vi "Multiprocessing_VI.vi"() -> ()   [LabVIEW 2022 SP3]
uses:
  <vilib>/Analysis/baseanly.llb/Mean (DBL).vi
  <vilib>/DAQmx/read.llb/DAQmx Read (Analog 1D Wfm NChan NSamp).vi
  STOP_GLOBAL.vi
  <vilib>/DAQmx/configure/timing.llb/DAQmx Timing (Sample Clock).vi
  <vilib>/addons/control/pid/pid.llb/PID Gain Schedule (DBL).vi
  <vilib>/DAQmx/miscellaneous.llb/DAQmx Fill In Error Info.vi
  <resource>/objmgr/daqmx.rc
  <vilib>/addons/control/pid/NI_PID_pid.lvlib
  <vilib>/Analysis/NI_AALBase.lvlib
panel:
  out "Angle Command":dynamicdata(graph)
  in  "Ignition":bool
  in  "Stepper Voltage":ext format="%_3g"
  out "Chamber Pressure LocalVar":dynamicdata(graph)
  out "PID gains out":T1={"proportional gain (Kc)"=1.0, "integral time (Ti, min)"=0.01, "derivative time (Td, min)"=0.0} {"derivative time (Td, min)" format="%.3f"; "integral time (Ti, min)" format="%.5f"; "proportional gain (Kc)" format="%.3f"}
  out "Process Variable vs Setpoint":dynamicdata(graph)
  out "Output":dbl(slide)=30.8641975308642 scale=0.0..5.067 scale format="%.1f"
  in  "Automatic":bool=TRUE
  out "Servo Voltage":dbl[](array[numeric])
  in  "SP":dbl
  in  "MV":dbl(slide)=30.8641975308642 scale=0.0..5.067 scale format="%.1f"
  in  "Stop All":bool
  out "x*y 2":dbl
  out "AI7":dynamicdata(graph)
  out "Time":dbl
  out "Inlet Thermocouple":cluster{dbl[], dbl[]}(graph)
  out "Inlet Thermocouple":dynamicdata(graph)
  out "Flow Meter Thermocouple":dynamicdata(graph)
  out "Supply P. Thermocouple":cluster{dbl[], dbl[]}(graph)
  out "Flow Meter Thermocouple":cluster{dbl[], dbl[]}(graph)
  out "Supply P. Thermocouple":dynamicdata(graph)
  out "Thrust 3":cluster{dbl[], dbl[]}(graph)
  out "Thrust 2":cluster{dbl[], dbl[]}(graph)
  out "Rocket Thrust":cluster{dbl[], dbl[]}(graph)
  out "LC3":dynamicdata(graph)
  out "LC2":dynamicdata(graph)
  out "Rocket Thrust LC1":dynamicdata(graph)
  out "Waiting \nfor Start":bool=TRUE
  in  "Start VI":bool
  out "SampClk.Rate":dbl
  in  "Sample Number":i32=100
  in  "Channel Control":bool[](array[boolean])
  in  "Rate":dbl=1000.0 format="%0.2f"
  out "AI7":cluster{dbl[], dbl[]}(graph)
  out "Vol Flow L/min":dynamicdata(graph)
  out "Process Variable vs Setpoint":cluster{dbl[], dbl[]}[](graph)
  in  "Filename":path=path "C:/1. Rocket Research Project/CollectedData/Plots/TestingData.lvm"
  in  "PID gain schedule":T2(array[cluster])=[{"PID gains"={"proportional gain (Kc)"=1.0, "integral time (Ti, min)"=0.01, "derivative time (Td, min)"=0.0}, "max value"=100.0}] {"max value" format="%.2f"; "PID gains"."derivative time (Td, min)" format="%.3f"; "PID gains"."integral time (Ti, min)" format="%.3f"; "PID gains"."proportional gain (Kc)" format="%.3f"}
  in  "Collect?":bool=TRUE caption="Enable"
  out "Vol Flow":cluster{dbl[], dbl[]}(graph)
  out "Chamber Pressure":cluster{dbl[], dbl[]}(graph)
  out "Inlet Pressure":cluster{dbl[], dbl[]}(graph)
  out "Line Pressure":cluster{dbl[], dbl[]}(graph)
  out "Supply Pressure":cluster{dbl[], dbl[]}(graph)
  out "Supply Pressure":dynamicdata(graph)
  out "Inlet Pressure":dynamicdata(graph)
  out "Line Pressure":dynamicdata(graph)
  out "Chamber Pressure PSI":dynamicdata(graph)
  out "Output Clock Rate":dbl
  out "x*y":i32
  out "error out":errorcluster
  out "Iterations":i32
  out "AI6":dynamicdata(graph)
  out "P.T. 5":dynamicdata(graph)
  # "Pressure Channels"
  # "Temperature Channels"
  # "Thrust Channels"
  # "DAQ Configuration"
  # "AI 0 - Supply Pressure"
  # "AI 1 - Flow Meter Pressure"
  # "AI 2 - Inlet Pressure"
  # "AI 3 - Chamber Pressure"
  # "AI 4 - Differential Pressure"
  # "AI 5 - Volumetric Flow"
  # "AI 6"
  # "AI 7"
  # "Load Cell 1 Right"
  # "Load Cell 2 Left"
  # "Thrust Channel 3"
  # "TC1 - Supply P. Thermocouple"
  # "TC2 - Flow Meter Thermocouple"
  # "TC3 - Inlet Thermocouple"
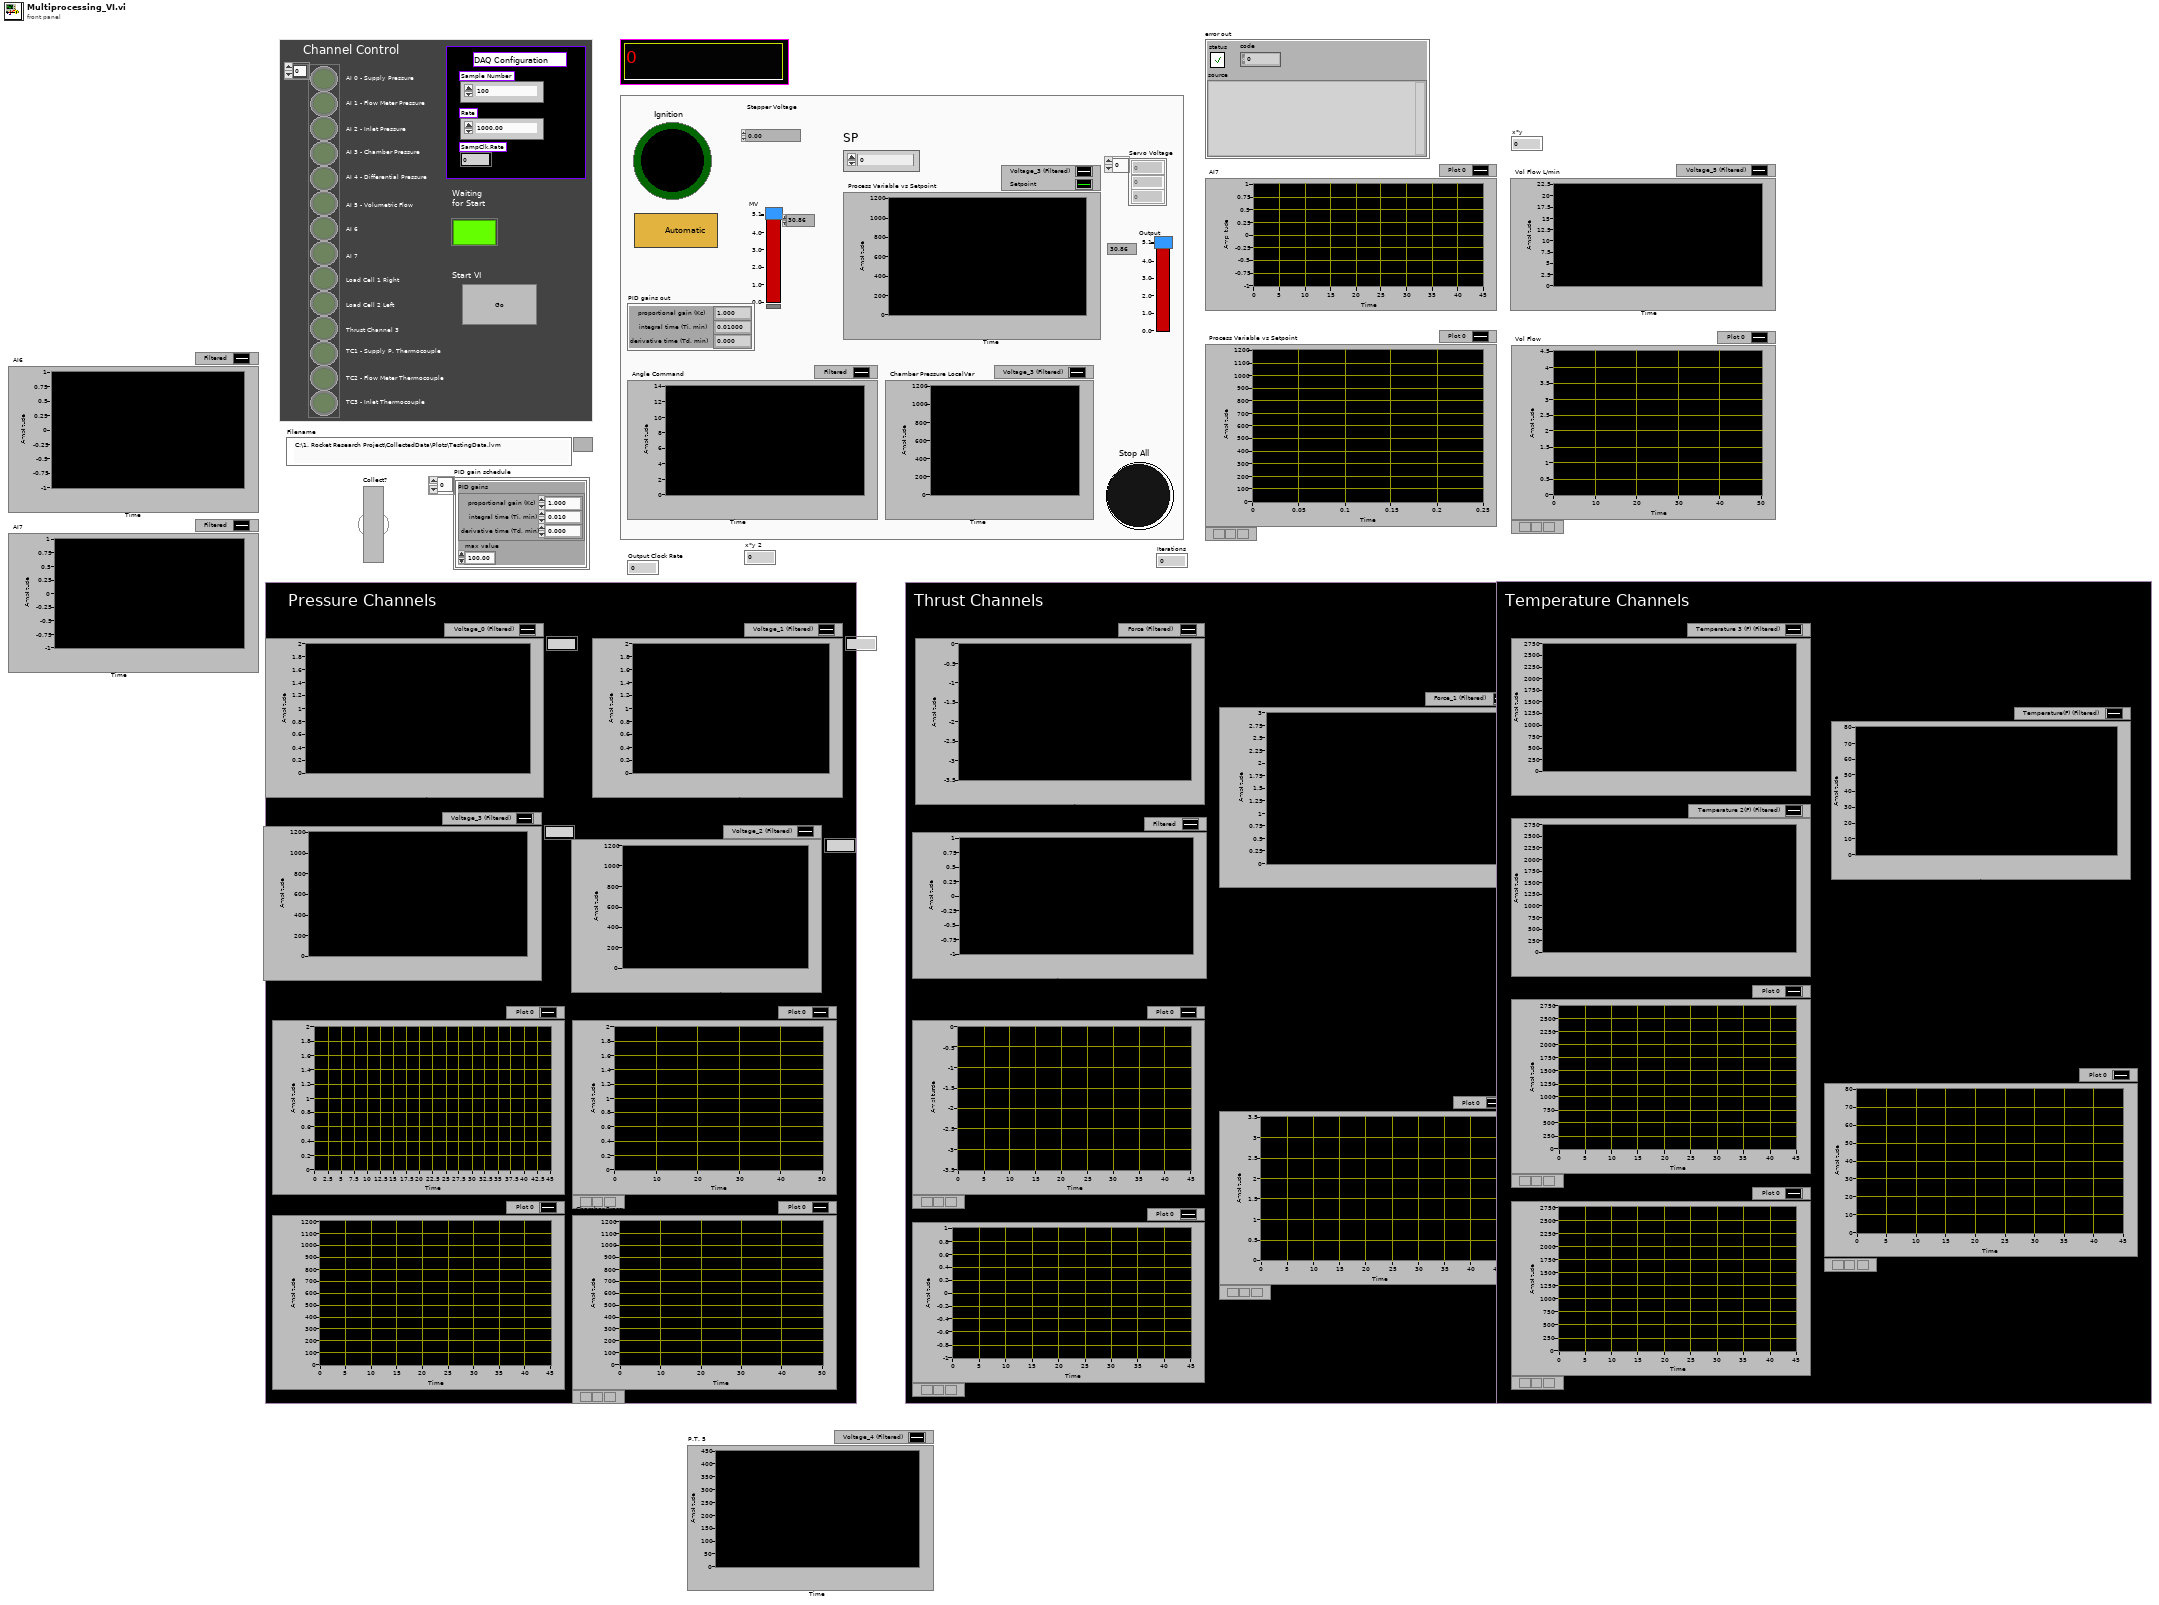
[diagram p1: front panel]
types:
  T1 = cluster{"proportional gain (Kc)":dbl, "integral time (Ti, min)":dbl, "derivative time (Td, min)":dbl}
  T2 = cluster{"PID gains":cluster{"proportional gain (Kc)":dbl, "integral time (Ti, min)":dbl, "derivative time (Td, min)":dbl}, "max value":dbl}[]
  T3 = cluster{"PID gains":cluster{"Kc":dbl, "Ti":dbl, "Td":dbl}, "max value":dbl}[]
  T4 = cluster{"Modulus":dbl, "Number of\nComplete Cycles":dbl}
  T5 = cluster{"Dynamic Data":dynamicdata, "Dynamic Data":dynamicdata, "Dynamic Data":dynamicdata, "Dynamic Data":dynamicdata, "Dynamic Data":dynamicdata, "Dynamic Data":dynamicdata, "Dynamic Data":dynamicdata, "Dynamic Data":dynamicdata, "Dynamic Data":dynamicdata, "Dynamic Data":dynamicdata, "Dynamic Data":dynamicdata, "Dynamic Data":dynamicdata, "Dynamic Data":dynamicdata, "Dynamic Data":dynamicdata}
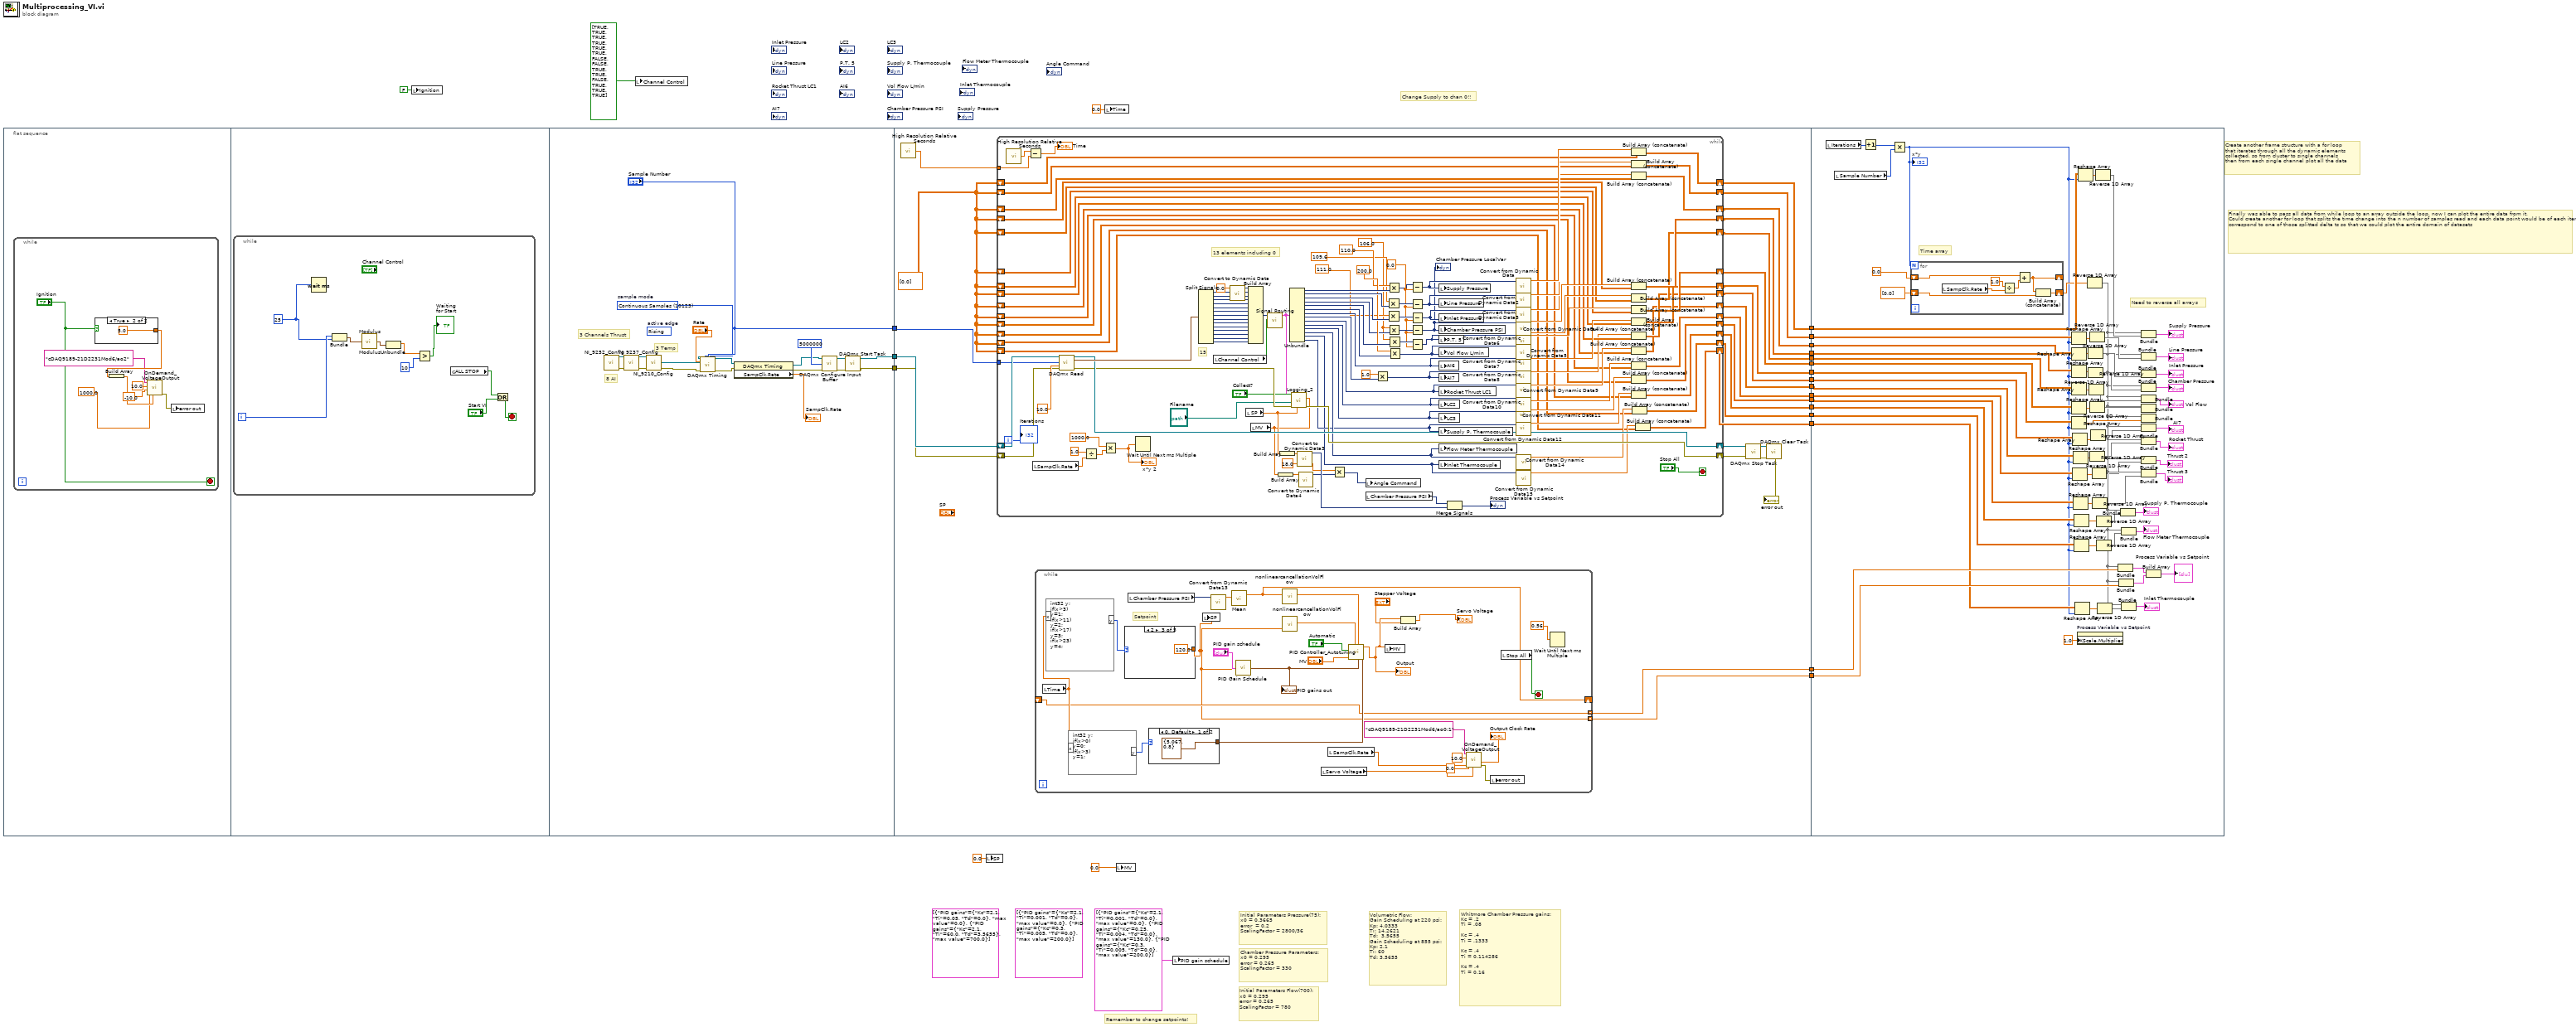
[diagram p0: block diagram]
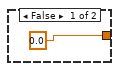
[diagram p2: hidden frame]
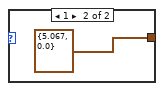
[diagram p3: hidden frame]
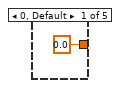
[diagram p4: hidden frame]
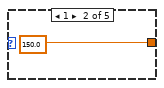
[diagram p5: hidden frame]
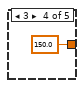
[diagram p6: hidden frame]
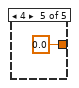
[diagram p7: hidden frame]
diagram:
  (unwired) T3 [{"PID gains"={"Kc"=2.1, "Ti"=0.05, "Td"=0.0}, "max value"=0.0}, {"PID gains"={"Kc"=2.1, "Ti"=60.0, "Td"=3.5655}, "max value"=700.0}]
  (unwired) T3 [{"PID gains"={"Kc"=2.1, "Ti"=0.001, "Td"=0.0}, "max value"=0.0}, {"PID gains"={"Kc"=0.3, "Ti"=0.005, "Td"=0.0}, "max value"=200.0}]
  # "Remember to change setpoints!"
  # "Whitmore Chamber Pressure gains:\nKc = .2\nTi = .08\n\nKc = .4\nTi = .1333\n\nKc = .4\nTi = 0.114286\n\nKc = .4\nTi = 0.16"
  # "Chamber Pressure Parameters:\nx0 = 0.295\nerror = 0.265\nScalingFactor = 330"
  # "Volumetric Flow:\nGain Scheduling at 220 psi:\nKp: 4.0333\nTi: 14.2621\nTd:  3.5655\nGain Scheduling at 855 psi:\nKp: 2.1\nTi: 60\nTd: 3.5655"
  # "Initial Parameters Flow(700):\nx0 = 0.295\nerror = 0.265\nScalingFactor = 780"
  # "Initial Parameters Pressure(75):\nx0 = 0.3665\nerror  = 0.2\nScalingFactor = 2800/36"
  # "Change Supply to chan 0!!"
  # "Finally was able to pass all data from while loop to an array outside the loop, now I can plot the entire data from it, \nCould create another for loop that splits the time change into the n number of samples read and each data point would be of each iteration would correspond to one of those splitted delta ts so that we could plot the entire domain of datasets"
  # "Create another frame structure with a for loop\nthat iterates through all the dynamic elements\ncollected, so from cluster to single channels\nthen from each single channel plot all the data"
  n1 = flat-sequence {
    tunnel: [w57] -> w24
    tunnel: [w46] -> w23
    tunnel: ["Sample Number"] -> w2
    tunnel: w24 -> [w90]
    tunnel: w23 -> [w89]
    tunnel: [w82] -> w22
    tunnel: [w81] -> w20
    tunnel: [w80] -> w19
    tunnel: [w79] -> w18
    tunnel: [w78] -> w17
    tunnel: [w77] -> w16
    tunnel: [w76] -> w15
    tunnel: [w75] -> w14
    tunnel: [w74] -> w13
    tunnel: [w73] -> w12
    tunnel: [w72] -> w11
    tunnel: [w71] -> w10
    tunnel: [w70] -> w8
    tunnel: [w69] -> w7
    tunnel: [w67] -> w4
    tunnel: [w66] -> w3
    tunnel: w2 -> [w65]
    tunnel: w22 -> [w310]
    tunnel: w20 -> [w309]
    tunnel: w19 -> [w308]
    tunnel: w18 -> [w307]
    tunnel: w17 -> [w306]
    tunnel: w16 -> [w305]
    tunnel: w15 -> [w304]
    tunnel: w14 -> [w302]
    tunnel: w13 -> [w301]
    tunnel: w12 -> [w300]
    tunnel: w11 -> [w299]
    tunnel: w10 -> [w298]
    tunnel: w8 -> [w293]
    tunnel: w7 -> [w292]
    tunnel: w4 -> [w267]
    tunnel: w3 -> [w266]
    frame #0 {
      n2 = while {
        stop <- "Ignition" stop-if-true
        n3 = case shown="True" "Ignition" {
          tunnel: [0.0 ("element") 5.0 ("element")] -> w32
          frame False {
          }
          frame True {
          }
        }
        n4 = Build Array(w32) -> (w33:dbl[])
        n5 = call "OnDemand_VoltageOutput.vi"("Channel Array"=w33, "SampClk.Rate 2"=1000.0, "minimum voltage"=-10.0, "maximum voltage"=10.0, "physical channels"="cDAQ9189-21D2231Mod6/ao2") -> ("error out"=w31:errorcluster)  [unwired: 4 in, 2 out]
        n6 = local write "error out"(w31) -> ()
      }
    }
    frame #1 {
      n7 = while {
        i -> [w45]
        stop <- w37 stop-if-true
        w36 = u32 25 ("milliseconds to wait")
        n8 = Wait (ms)(milliseconds to wait=w36) -> ()  [unwired: 1 out]
        n9 = Bundle(w45, "milliseconds to wait"=w36) -> (w44:cluster{i32, "milliseconds to wait":u32})  [unwired: 1 in]
        n10 = call "Modulus.vi"("Input"=w44) -> ("Output"=w43:T4)
        n11 = call "Modulus.vi"() -> ()  [unwired: 1 in, 1 out]
        n12 = Unbundle(w43) -> ("Modulus"=w42:dbl)  [unwired: 1 out]
        n13 = Greater?(x=w42, y=u32 10 ("milliseconds to wait")) -> (0:→"Waiting \nfor Start":bool)
        n14 = global read "STOP_GLOBAL.vi" "ALL STOP"() -> (w39:bool)
        n15 = Or(x=w39, y="Start VI") -> (x .or. y?=w37:bool)
      }
    }
    frame #2 {
      w48 = 10123 items=["Finite Samples"=10178, "Continuous Samples"=10123, "Hardware Timed Single Point"=12522]  # sample mode
      (unwired) 10280 items=["Rising"=10280, "Falling"=10171]  # active edge
      # "3 Temp"
      # "8 AI"
      # "3 Channels Thrust"
      n16 = call "NI_9252_Config.vi"() -> ("error out"=w55:errorcluster, "task out"=w56:refnum<k21>)  [unwired: 10 in]
      n17 = call "NI 9237_Config.vi"("error in"=w55, "task in"=w56) -> ("error out"=w64:errorcluster, "task out"=w63:refnum<k21>)  [unwired: 8 in]
      n18 = call "NI_9210_Config.vi"("error in"=w64, "task in"=w63) -> ("error out"=w51:errorcluster, "task out"=w53:refnum<k21>)  [unwired: 8 in]
      n19 = call-poly <vilib>:"DAQmx Timing.vi"("task/channels in"=w53, "sample mode"=w48, "samples per channel"="Sample Number", "rate"="Rate", "error in"=w51) -> ("task out"=w49:refnum<k21>, "error out"=w50:errorcluster)  [unwired: 9 in]
      n20 = property class="DAQmx Timing"(reference=w49, error in=w50) -> (reference out=w47:refnum<k21>, error out=w60:errorcluster, "SampClk.Rate"=→"SampClk.Rate":dbl)
      n21 = call <vilib>:"DAQmx Configure Input Buffer.vi"("task/channels in"=w47, "buffer size (in samples per channel)"=u32 5000000, "error in"=w60) -> ("task out"=w62:refnum<k21>, "error out"=w61:errorcluster)  [unwired: 11 in]
      n22 = call <vilib>:"DAQmx Start Task.vi"("task/channels in"=w62, "error in"=w61) -> ("task out"=w57:refnum<k21>, "error out"=w46:errorcluster)  [unwired: 12 in]
    }
    frame #3 {
      w68 = dbl[][] [[0.0]]
      n23 = call <vilib>:"High Resolution Relative Seconds.vi"() -> ("relative seconds"=w88:dbl)
      n24 = while {
        shift-right: [w244] -> w84
        shift-left: w90 -> [w246]
        shift-right: [w222] -> w83
        shift-left: w89 -> [w245]
        shift-right: [w125] -> w82
        shift-left: w68 -> [w178]
        tunnel: w88 -> [w218]
        shift-right: [w212] -> w81
        shift-left: w68 -> [w213]
        shift-right: [w208] -> w80
        shift-left: w68 -> [w209]
        shift-right: [w206] -> w79
        shift-left: w68 -> [w207]
        shift-right: [w204] -> w78
        shift-left: w68 -> [w203]
        shift-right: [w200] -> w77
        shift-left: w68 -> [w198]
        shift-right: [w199] -> w76
        shift-left: w68 -> [w197]
        shift-right: [w196] -> w75
        shift-left: w68 -> [w195]
        shift-right: [w189] -> w74
        shift-left: w68 -> [w188]
        shift-right: [w187] -> w73
        shift-left: w68 -> [w186]
        shift-right: [w183] -> w72
        shift-left: w68 -> [w182]
        shift-right: [w180] -> w71
        shift-left: w68 -> [w179]
        shift-right: [w157] -> w67
        shift-left: w68 -> [w156]
        shift-right: [w153] -> w66
        shift-left: w68 -> [w154]
        tunnel: w65 -> [w150]
        i -> [w220]
        stop <- "Stop All" stop-if-true
        w126 = 106.0 ("x")
        w141 = 0.0 ("y")
        # "13 elements including 0"
        # "15"
        n25 = call <vilib>:"High Resolution Relative Seconds.vi"() -> ("relative seconds"=w219:dbl)
        n26 = Subtract(x=w219, y=w218) -> (x-y=→"Time":dbl)
        n27 = local read "SampClk.Rate"() -> (w175:dbl)
        n28 = call-poly <vilib>:"DAQmx Read.vi"("task/channels in"=w246, "number of samples per channel"=w150, "timeout"=10.0, "error in"=w245) -> ("task out"=w244:refnum<k21>, "data"=w247:waveform(dbl)[], "error out"=w224:errorcluster)  [unwired: 9 in]
        n29 = Divide(x=1.0, y=w175) -> (x/y=w174:dbl)
        n30 = Multiply(x=1000.0, y=w174) -> (x*y=w172:dbl)
        "x*y 2" <- w172
        n31 = Wait Until Next ms Multiple(millisecond multiple=w172) -> ()  [unwired: 1 out]
        n32 = Split Signals(w247) -> (w238:dynamicdata, w243:dynamicdata, w242:dynamicdata, w241:dynamicdata, w240:dynamicdata, w239:dynamicdata, w237:dynamicdata, w236:dynamicdata, w235:dynamicdata, w234:dynamicdata, w233:dynamicdata, w230:dynamicdata, w160:dynamicdata, w159:dynamicdata)  [unwired: 14 in]
        n33 = local read "Channel Control"() -> (w229:bool[])
        n34 = call "Convert to Dynamic Data"("Double"=0.0) -> ("Dynamic Data Type"=w231:dynamicdata)  [unwired: 3 in]
        n35 = local read "SP"() -> (w139:dbl)
        n36 = Build Array(w231, w238, w243, w242, w241, w240, w239, w237, w236, w235, w234, w233, w230, w160, w159) -> (w228:dynamicdata[])
        n37 = local read "MV"() -> (w134:dbl)
        n38 = call "Signal Routing.vi"("Boolean Array"=w229, "Data In"=w228) -> ("Output"=w149:T5)  [unwired: 9 in]
        n39 = Build Array(w134) -> (w133:dbl[])
        n40 = Build Array(w139) -> (w138:dbl[])
        n41 = Unbundle(w149) -> ("Dynamic Data"=w221:dynamicdata, "Dynamic Data"=w227:dynamicdata, "Dynamic Data"=w226:dynamicdata, "Dynamic Data"=w140:dynamicdata, "Dynamic Data"=w225:dynamicdata, "Dynamic Data"=w152:dynamicdata, "Dynamic Data"=w144:dynamicdata, "Dynamic Data"=w171:dynamicdata, "Dynamic Data"=w194:dynamicdata, "Dynamic Data"=w190:dynamicdata, "Dynamic Data"=w185:dynamicdata, "Dynamic Data"=w148:dynamicdata, "Dynamic Data"=w146:dynamicdata, "Dynamic Data"=w147:dynamicdata)
        n42 = call "Logging_2.vi"("Voltage Command"=w134, "Setpoint"=w139, "error in"=w224, "Filename"="Filename", "Enable"="Collect?", "output cluster"=w149) -> ("error out"=w222:errorcluster)  [unwired: 5 in]
        n43 = call "Convert to Dynamic Data3"("Array"=w138) -> ("Dynamic Data Type"=w137:dynamicdata)  [unwired: 3 in]
        n44 = call "Convert to Dynamic Data4"("Array"=w133) -> ("Dynamic Data Type"=w132:dynamicdata)  [unwired: 3 in]
        n45 = Multiply(x=18.0, y=w132) -> (x*y=w130:dynamicdata)
        n46 = local write "Angle Command"(w130) -> ()
        n47 = local read "Chamber Pressure PSI"() -> (w135:dynamicdata)
        n48 = Multiply(x=1.0, y=w171) -> (x*y=w169:dynamicdata)
        n49 = Multiply(x=109.6, y=w227) -> (x*y=w167:dynamicdata)
        n50 = Multiply(x=111.0, y=w226) -> (x*y=w168:dynamicdata)
        n51 = Multiply(x=110.0, y=w221) -> (x*y=w166:dynamicdata)
        n52 = Multiply(x=w126, y=w140) -> (x*y=w162:dynamicdata)
        n53 = Multiply(x=w126, y=w225) -> (x*y=w143:dynamicdata)
        n54 = Multiply(x=200.0, y=w152) -> (x*y=w145:dynamicdata)
        n55 = Subtract(x=w166, y=w141) -> (x-y=w165:dynamicdata)
        n56 = Subtract(x=w167, y=w141) -> (x-y=w164:dynamicdata)
        n57 = Subtract(x=w168, y=w141) -> (x-y=w163:dynamicdata)
        n58 = Subtract(x=w162, y=w141) -> (x-y=w161:dynamicdata)
        "Chamber Pressure LocalVar" <- w161
        n59 = Subtract(x=w143, y=w141) -> (x-y=w142:dynamicdata)
        n60 = local write "Supply Pressure"(w165) -> ()
        n61 = local write "Line Pressure"(w164) -> ()
        n62 = local write "Inlet Pressure"(w163) -> ()
        n63 = local write "Chamber Pressure PSI"(w161) -> ()
        n64 = local write "P.T. 5"(w142) -> ()
        n65 = local write "Vol Flow L/min"(w145) -> ()
        n66 = local write "AI6"(w144) -> ()
        n67 = local write "AI7"(w169) -> ()
        n68 = local write "Rocket Thrust LC1"(w194) -> ()
        n69 = local write "LC2"(w190) -> ()
        n70 = local write "LC3"(w185) -> ()
        n71 = local write "Supply P. Thermocouple"(w147) -> ()
        n72 = local write "Flow Meter Thermocouple"(w148) -> ()
        n73 = local write "Inlet Thermocouple"(w146) -> ()
        n74 = Merge Signals(w135, w137) -> (→"Process Variable vs Setpoint":dynamicdata)
        n75 = call "Convert from Dynamic Data"("Dynamic Data Type"=w165) -> ("Array"=w217:dbl[])  [unwired: 3 in]
        n76 = call "Convert from Dynamic Data2"("Dynamic Data Type"=w164) -> ("Array"=w214:dbl[])  [unwired: 3 in]
        n77 = call "Convert from Dynamic Data3"("Dynamic Data Type"=w163) -> ("Array"=w211:dbl[])  [unwired: 3 in]
        n78 = call "Convert from Dynamic Data4"("Dynamic Data Type"=w161) -> ("Array"=w210:dbl[])  [unwired: 3 in]
        n79 = call "Convert from Dynamic Data6"("Dynamic Data Type"=w142) -> ("Array"=w202:dbl[])  [unwired: 3 in]
        n80 = call "Convert from Dynamic Data5"("Dynamic Data Type"=w145) -> ("Array"=w205:dbl[])  [unwired: 3 in]
        n81 = call "Convert from Dynamic Data7"("Dynamic Data Type"=w144) -> ("Array"=w201:dbl[])  [unwired: 3 in]
        n82 = call "Convert from Dynamic Data8"("Dynamic Data Type"=w169) -> ("Array"=w193:dbl[])  [unwired: 3 in]
        n83 = call "Convert from Dynamic Data9"("Dynamic Data Type"=w194) -> ("Array"=w192:dbl[])  [unwired: 3 in]
        n84 = call "Convert from Dynamic Data10"("Dynamic Data Type"=w190) -> ("Array"=w191:dbl[])  [unwired: 3 in]
        n85 = call "Convert from Dynamic Data11"("Dynamic Data Type"=w185) -> ("Array"=w184:dbl[])  [unwired: 3 in]
        n86 = call "Convert from Dynamic Data12"("Dynamic Data Type"=w147) -> ("Array"=w181:dbl[])  [unwired: 3 in]
        n87 = call "Convert from Dynamic Data14"("Dynamic Data Type"=w148) -> ("Array"=w158:dbl[])  [unwired: 3 in]
        n88 = call "Convert from Dynamic Data15"("Dynamic Data Type"=w146) -> ("Array"=w155:dbl[])  [unwired: 3 in]
        n89 = Build Array (concatenate)(w217, w178) -> (w125:dbl[][])
        n90 = Build Array (concatenate)(w214, w213) -> (w212:dbl[][])
        n91 = Build Array (concatenate)(w211, w209) -> (w208:dbl[][])
        n92 = Build Array (concatenate)(w210, w207) -> (w206:dbl[][])
        n93 = Build Array (concatenate)(w205, w203) -> (w204:dbl[][])
        n94 = Build Array (concatenate)(w202, w198) -> (w200:dbl[][])
        n95 = Build Array (concatenate)(w201, w197) -> (w199:dbl[][])
        n96 = Build Array (concatenate)(w193, w195) -> (w196:dbl[][])
        n97 = Build Array (concatenate)(w192, w188) -> (w189:dbl[][])
        n98 = Build Array (concatenate)(w191, w186) -> (w187:dbl[][])
        n99 = Build Array (concatenate)(w184, w182) -> (w183:dbl[][])
        n100 = Build Array (concatenate)(w181, w179) -> (w180:dbl[][])
        n101 = Build Array (concatenate)(w158, w156) -> (w157:dbl[][])
        n102 = Build Array (concatenate)(w155, w154) -> (w153:dbl[][])
        "Iterations" <- w220
      }
      n103 = while {
        shift-right: [w108] -> _
        shift-left: _ -> [w103]
        tunnel: [w103] -> w70 mode=indexing
        tunnel: [w94] -> w69 mode=indexing
        stop <- w111 stop-if-true
        # "Setpoint"
        n104 = local read "Time"() -> (w106:dbl)
        n105 = formula code="int32 y;\nif(x>3)\ny=1;\nif(x>11)\ny=2;\nif(x>17)\ny=3;\nif(x>23)\ny=4;"("x"=w106) -> ("y"=w107:i32)
        n106 = formula code="int32 y;\nif(x>0)\ny=0;\nif(x>3)\ny=1;"("x"=w106) -> ("y"=w105:i32)
        n107 = case shown="2" w107 {
          tunnel: [0.0 ("SP") 150.0 ("SP") 120.0 ("SP") 150.0 ("SP") 0.0 ("SP")] -> w94
          frame 0, Default {
          }
          frame 1 {
          }
          frame 2 {
          }
          frame 3 {
          }
          frame 4 {
          }
        }
        n108 = local read "Chamber Pressure PSI"() -> (w92:dynamicdata)
        n109 = case shown="0, Default" w105 {
          tunnel: [cluster{"output high":dbl, "output low":dbl} {"output high"=5.067, "output low"=0.8} ("output range") cluster{"output high":dbl, "output low":dbl} {"output high"=5.067, "output low"=0.0} ("output range")] -> w104
          frame 0, Default {
          }
          frame 1 {
          }
        }
        n110 = local write "SP"(w94) -> ()
        n111 = call "Convert from Dynamic Data13"("Dynamic Data Type"=w92) -> ("Array"=w109:dbl[])  [unwired: 3 in]
        n112 = call-poly <vilib>:"Mean.vi"("X"=w109) -> ("mean"=w108:dbl)  [unwired: 1 out]
        n113 = call-poly <vilib>:"PID Gain Schedule.vi"("PID gain schedule"="PID gain schedule", "gain scheduling value"=w94) -> ("PID gains out"=w116:T1)  [unwired: 2 in, 1 out]
        "PID gains out" <- w116
        n114 = call "nonlinearcancellationVolFlow.vi"("input variable"=w108) -> ("MVT Process Variable"=w110:dbl)  [unwired: 10 in]
        n115 = call "nonlinearcancellationVolFlow.vi"("input variable"=w94) -> ("MVT Process Variable"=w114:dbl)  [unwired: 10 in]
        n116 = local read "Servo Voltage"() -> (w100:dbl[])
        n117 = local read "SampClk.Rate"() -> (w101:dbl)
        n118 = call "PID Controller_Autotuning.vi"("output range"=w104, "PID gains in"=w116, "process variable"=w110, "setpoint"=w114, "manipulated variable"="MV", "Automatic"="Automatic") -> ("output"=w112:dbl)  [unwired: 4 in, 1 out]
        "Output" <- w112
        n119 = local write "MV"(w112) -> ()
        n120 = Build Array(w112, "Stepper Voltage") -> (→"Servo Voltage":ext[])
        n121 = call "OnDemand_VoltageOutput.vi"("Channel Array"=w100, "SampClk.Rate 2"=w101, "minimum voltage"=0.0, "maximum voltage"=10.0, "physical channels"="cDAQ9189-21D2231Mod6/ao0:1") -> ("error out"=w99:errorcluster, "SampClk.Rate"=→"Output Clock Rate":dbl)  [unwired: 4 in, 1 out]
        n122 = local write "error out"(w99) -> ()
        n123 = local read "Stop All"() -> (w111:bool)
        n124 = Wait Until Next ms Multiple(millisecond multiple=0.56 ("x")) -> ()  [unwired: 1 out]
      }
      n125 = call <vilib>:"DAQmx Stop Task.vi"("task/channels in"=w84, "error in"=w83) -> ("task out"=w87:refnum<k21>, "error out"=w86:errorcluster)  [unwired: 12 in]
      n126 = call <vilib>:"DAQmx Clear Task.vi"("task in"=w87, "error in"=w86) -> ("error out"=→"error out":errorcluster)  [unwired: 13 in]
    }
    frame #4 {
      # "Time array"
      # "Need to reverse all arrays"
      n127 = local read "Iterations"() -> (w315:i32)
      n128 = local read "Sample Number"() -> (w249:i32)
      n129 = Increment(x=w315) -> (x+1=w314:i32)
      n130 = Multiply(x=w314, y=w249) -> (x*y=w265:i32)
      "x*y" <- w265
      n131 = for {
        N: w265 -> [_]
        shift-right: [w318] -> _
        shift-left: 0.0 -> [w319]
        shift-right: [w317] -> w288
        shift-left: dbl[] [0.0] -> [w316]
        n132 = local read "SampClk.Rate"() -> (w321:dbl)
        n133 = Divide(x=1.0, y=w321) -> (x/y=w320:dbl)
        n134 = Add(x=w319, y=w320) -> (x+y=w318:dbl)
        n135 = Build Array (concatenate)(w318, w316) -> (w317:dbl[])
      }
      n136 = Reshape Array(w309, w265) -> (w284:dbl[])
      n137 = Reshape Array(w308, w265) -> (w282:dbl[])
      n138 = Reshape Array(w307, w265) -> (w280:dbl[])
      n139 = Reshape Array(w306, w265) -> (w278:dbl[])
      n140 = Reshape Array(w305, w265) -> (w276:dbl[])
      n141 = Reshape Array(w304, w265) -> (w303:dbl[])
      n142 = Reshape Array(w302, w265) -> (w273:dbl[])
      n143 = Reshape Array(w300, w265) -> (w255:dbl[])
      n144 = Reshape Array(w301, w265) -> (w264:dbl[])
      n145 = Reshape Array(w299, w265) -> (w252:dbl[])
      n146 = Reshape Array(w298, w265) -> (w270:dbl[])
      n147 = Reshape Array(w267, w265) -> (w262:dbl[])
      n148 = Reshape Array(w266, w265) -> (w256:dbl[])
      n149 = property on="Process Variable vs Setpoint" class="XYGraph (strict)"("XScale.Multiplier"=1.0 ("X Scale.Offset and Multiplier:Multiplier")) -> ()  [unwired: 2 in, 2 out]
      n150 = Reshape Array(w310, w265) -> (w286:dbl[])
      n151 = Reverse 1D Array(array=w288) -> (reversed array=w259:dbl[])
      n152 = Reverse 1D Array(array=w282) -> (reversed array=w281:dbl[])
      n153 = Reverse 1D Array(array=w280) -> (reversed array=w279:dbl[])
      n154 = Reverse 1D Array(array=w278) -> (reversed array=w277:dbl[])
      n155 = Reverse 1D Array(array=w284) -> (reversed array=w283:dbl[])
      n156 = Reverse 1D Array(array=w276) -> (reversed array=w275:dbl[])
      n157 = Reverse 1D Array(array=w264) -> (reversed array=w263:dbl[])
      n158 = Reverse 1D Array(array=w273) -> (reversed array=w272:dbl[])
      n159 = Reverse 1D Array(array=w255) -> (reversed array=w254:dbl[])
      n160 = Reverse 1D Array(array=w252) -> (reversed array=w251:dbl[])
      n161 = Reverse 1D Array(array=w286) -> (reversed array=w285:dbl[])
      n162 = Reverse 1D Array(array=w270) -> (reversed array=w269:dbl[])
      n163 = Reverse 1D Array(array=w262) -> (reversed array=w261:dbl[])
      n164 = Reverse 1D Array(array=w256) -> (reversed array=w257:dbl[])
      n165 = Bundle(w259, w293) -> (w290:cluster{dbl[], dbl[]})  [unwired: 1 in]
      n166 = Bundle(w259, w292) -> (w291:cluster{dbl[], dbl[]})  [unwired: 1 in]
      n167 = Bundle(w259, w269) -> (→"Supply P. Thermocouple":cluster{dbl[], dbl[]})  [unwired: 1 in]
      n168 = Bundle(w259, w261) -> (→"Flow Meter Thermocouple":cluster{dbl[], dbl[]})  [unwired: 1 in]
      n169 = Bundle(w259, w257) -> (→"Inlet Thermocouple":cluster{dbl[], dbl[]})  [unwired: 1 in]
      n170 = Bundle(w259, w285) -> (→"Supply Pressure":cluster{dbl[], dbl[]})  [unwired: 1 in]
      n171 = Bundle(w259, w283) -> (→"Line Pressure":cluster{dbl[], dbl[]})  [unwired: 1 in]
      n172 = Bundle(w259, w281) -> (→"Inlet Pressure":cluster{dbl[], dbl[]})  [unwired: 1 in]
      n173 = Bundle(w259, w279) -> (→"Chamber Pressure":cluster{dbl[], dbl[]})  [unwired: 1 in]
      n174 = Bundle(w259, w277) -> (→"Vol Flow":cluster{dbl[], dbl[]})  [unwired: 1 in]
      n175 = Bundle(w259, w275) -> ()  [unwired: 1 in, 1 out]
      n176 = Bundle(w259, w303) -> ()  [unwired: 1 in, 1 out]
      n177 = Bundle(w259, w272) -> (→"AI7":cluster{dbl[], dbl[]})  [unwired: 1 in]
      n178 = Bundle(w259, w263) -> (→"Rocket Thrust":cluster{dbl[], dbl[]})  [unwired: 1 in]
      n179 = Bundle(w259, w254) -> (→"Thrust 2":cluster{dbl[], dbl[]})  [unwired: 1 in]
      n180 = Bundle(w259, w251) -> (→"Thrust 3":cluster{dbl[], dbl[]})  [unwired: 1 in]
      n181 = Build Array(w290, w291) -> (→"Process Variable vs Setpoint":cluster{dbl[], dbl[]}[])
    }
  }
  n182 = local write "Ignition"(FALSE ("Ignition")) -> ()
  n183 = local write "Channel Control"(bool[] [TRUE, TRUE, TRUE, TRUE, TRUE, TRUE, FALSE, FALSE, TRUE, TRUE, FALSE, TRUE, TRUE, TRUE] ("Array")) -> ()
  n184 = local write "SP"(0.0 ("SP")) -> ()
  n185 = local write "Time"(0.0 ("Time")) -> ()
  n186 = local write "MV"(0.0 ("MV")) -> ()
  n187 = local write "PID gain schedule"(T3 [{"PID gains"={"Kc"=2.1, "Ti"=0.001, "Td"=0.0}, "max value"=0.0}, {"PID gains"={"Kc"=0.25, "Ti"=0.004, "Td"=0.0}, "max value"=130.0}, {"PID gains"={"Kc"=0.3, "Ti"=0.005, "Td"=0.0}, "max value"=200.0}]) -> ()
